vi "图像采集与保存-简单图像处理(加录像功能).vi"(9 "Grab":bool, 11 "Camera Name":refnum<k21>="cam0" caption="IMAQdx Session") -> ()   [LabVIEW 2022 SP3]
doc: "The Grab and Attributes Setup example VI allows the user to view the current attributes and settings, update attribute settings, acquire images continuously, and display the images in an image control."
uses:
  <vilib>/vision/Avi.llb/IMAQ AVI2 Refnum.ctl
  <vilib>/vision/driver/IMAQdx.llb/IMAQdx Acquisition Mode.ctl
  <vilib>/vision/driver/IMAQdx.llb/IMAQdx Buffer Number Mode.ctl
  <vilib>/vision/driver/NI_Vision_Acquisition_Software.lvlib
panel:
  in  "Boolean":bool
  out "视频路径":path
  out "time":u32
  out "Image 2":T1(plugin-control)
  out "AVI Refnum (duplicate)":T2
  out "millisecond timer value":u32
  out "AVI Refnum":T2
  in  "录制视频":bool
  out "Image out":T1(plugin-control)
  out "错误输出":errorcluster
  out "返回值":i32
  out "处理图片路径":path
  out "采集图片路径":path
  out "帧数":i32
  in  "采集帧间隔":i8
  in  "确定按钮":bool
  in  "Tab Control":T3(tab)
  in  "U32 Value Control":u32(slide) min=1 step=1 scale=1.0..4294967295.0
  in  "DBL Value Control":dbl(slide) min=2.2571161239684447 max=1000.0 step=1.0 scale=2.2571161239684447..1000.0
  in  "String Value Control":string
  in  "Enum Value Control":u32(ring) items=["Unicast", "Broadcast", "Multicast"]
  in  "Boolean Value Control":bool
  in  "Command Value Control":bool
  out "Tooltip":string="Gets/Sets the maximum number of outstanding events to queue."
  out "Units":string
  in  "Attribute Tree":string(tree)
  out "Frame Rate":dbl(knob) scale=0.0..100.0
  out "Image":T1(plugin-control)
  out "Buffer Number":u32
  in  "Stop":bool
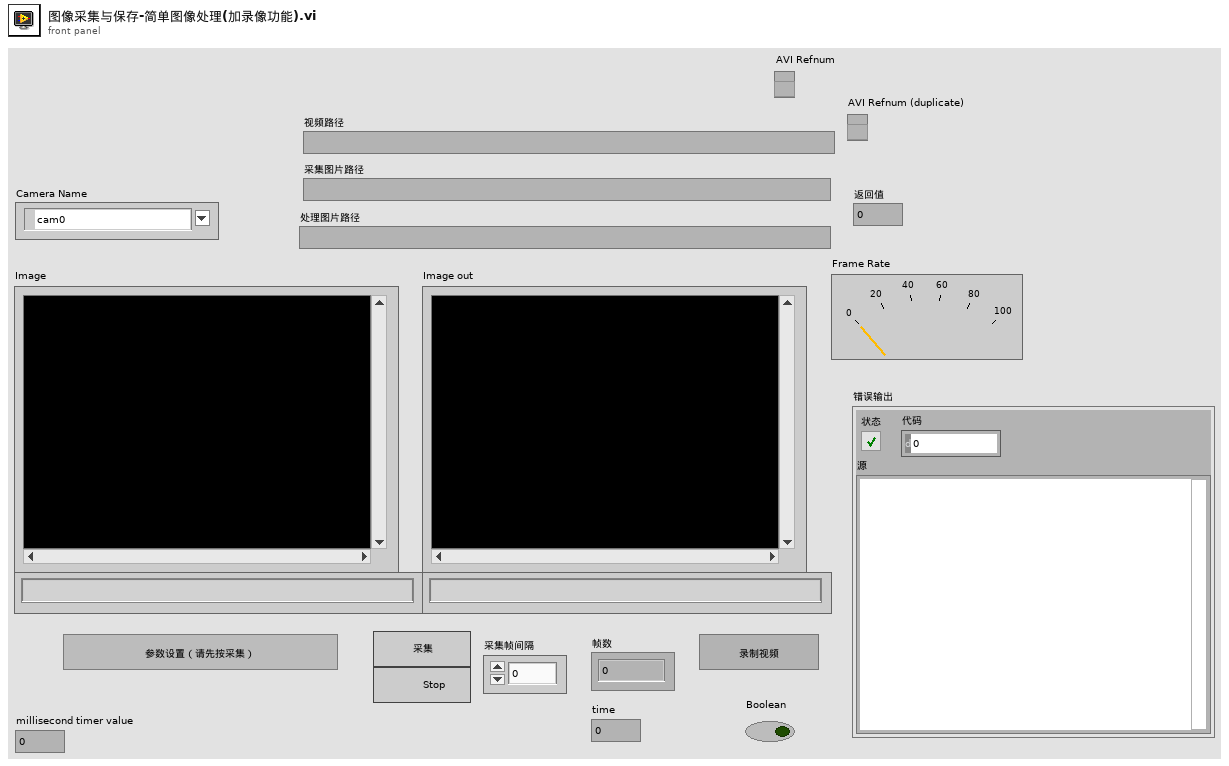
[diagram p1: front panel]
types:
  T1 = typedef "IMAQ Image.ctl" = refnum<image>
  T2 = typedef "IMAQ AVI2 Refnum.ctl" = refnum<k20>
  T3 = enum32{"U32", "DBL", "String", "Enum", "Bool", "Command"}
  T4 = typedef "NI_Vision_Acquisition_Software.lvlib/IMAQdx Acquisition Mode.ctl" = enum32{"One Shot", "Continuous"}
  T5 = typedef "IMAQdx.ctl" = refnum<k21>
  T6 = cluster{"Tab Control":refnum<vi>, "U32 Value Control":refnum<vi>, "DBL Value Control":refnum<vi>, "String Value Control":refnum<vi>, "Enum Value Control":refnum<vi>, "Boolean Value Control":refnum<vi>, "Command Value Control":refnum<vi>}
  T7 = typedef "NI_Vision_Acquisition_Software.lvlib/IMAQdx Buffer Number Mode.ctl" = enum32{"Next", "Last", "Buffer Number", "Every", "Last New"}
  T8 = typedef "Image Type" = u32
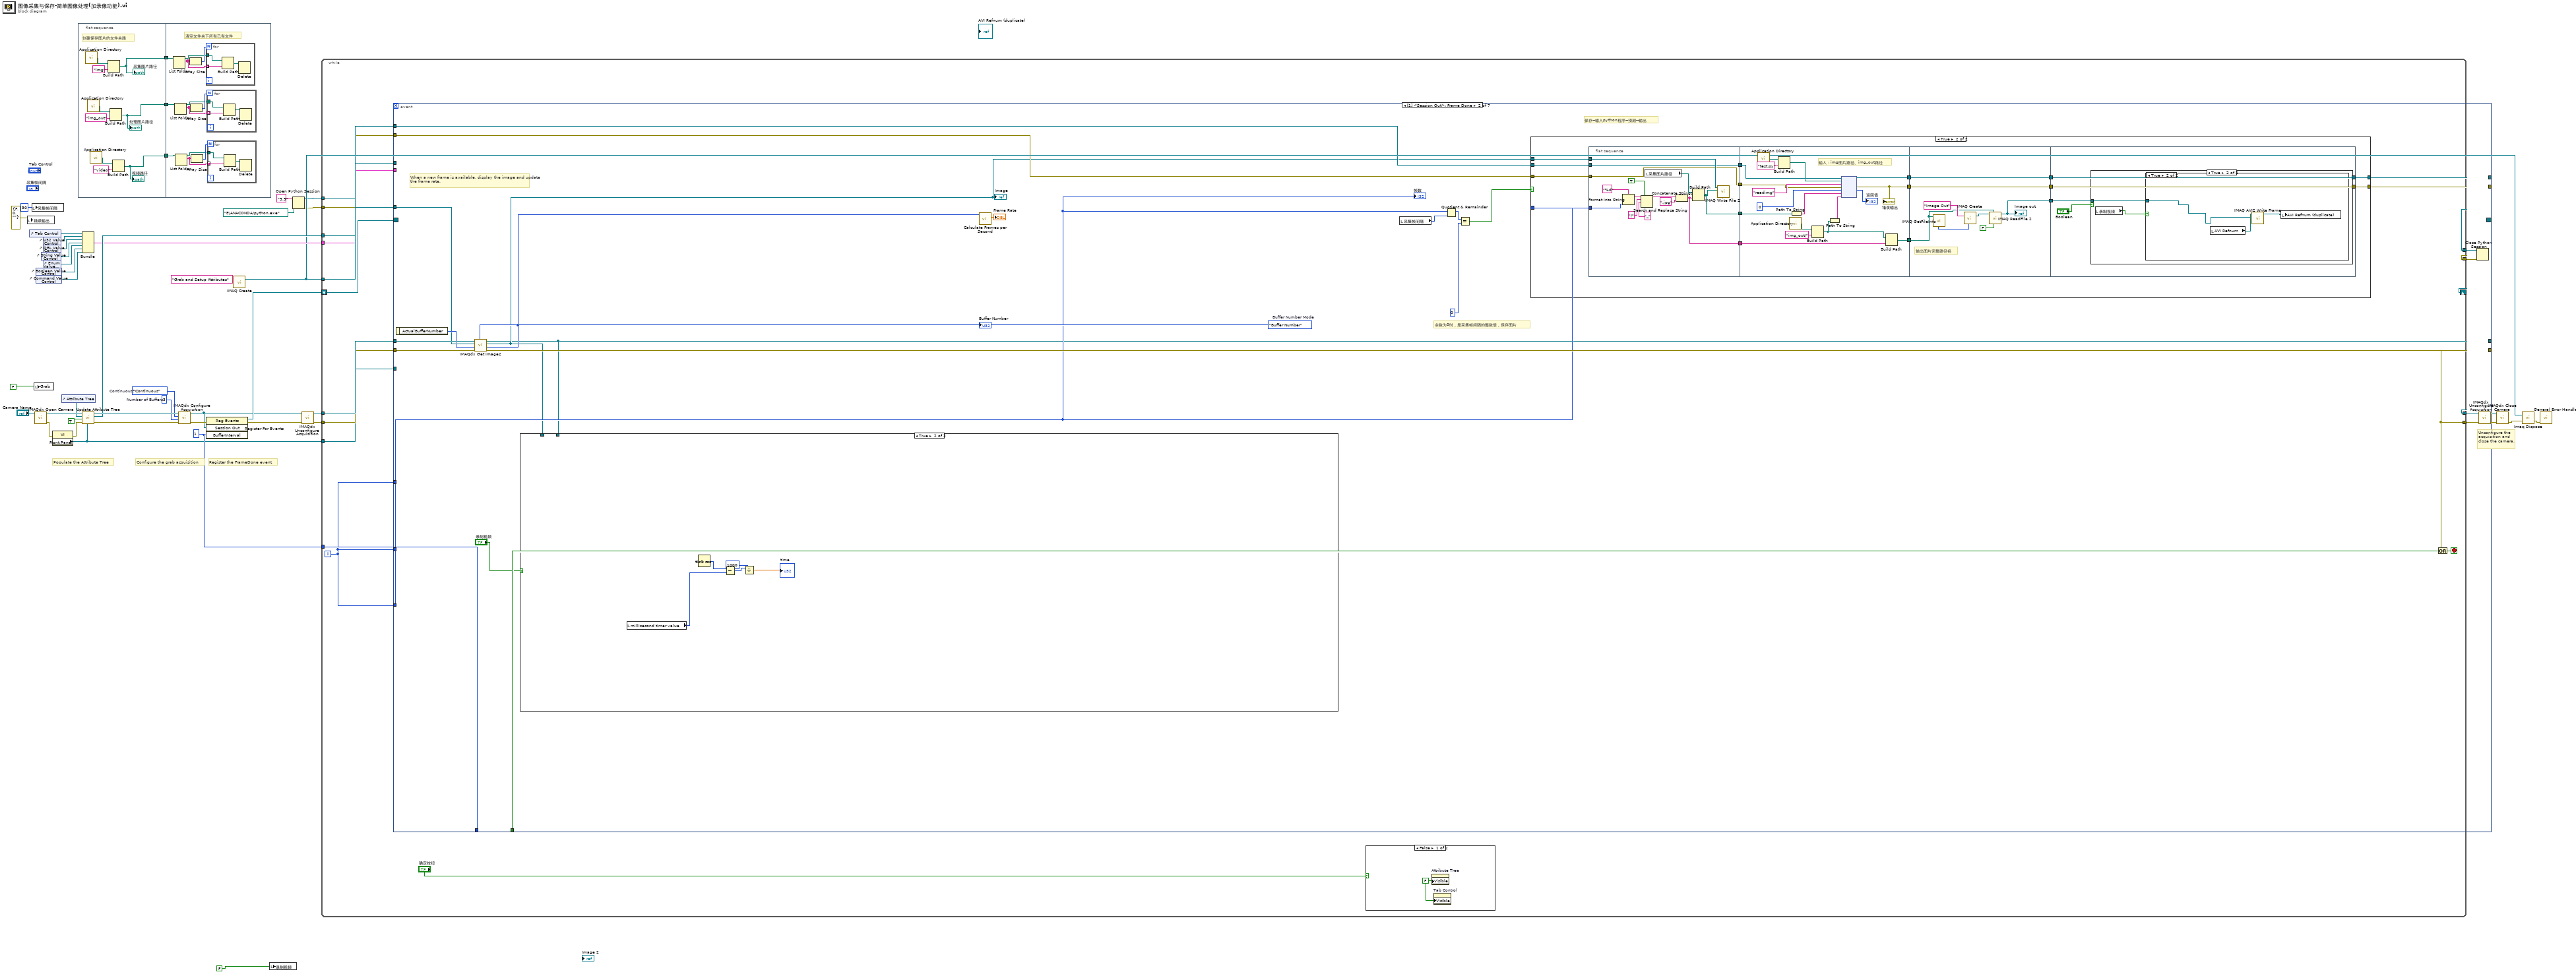
[diagram p0: block diagram]
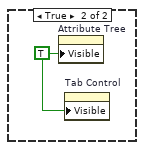
[diagram p2: hidden frame]
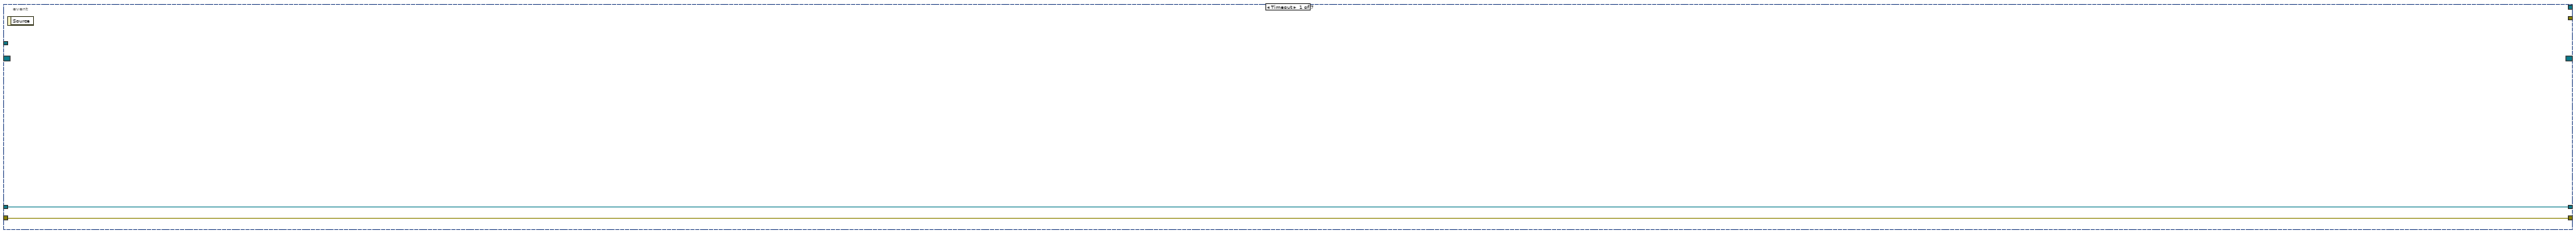
[diagram p3: hidden frame]
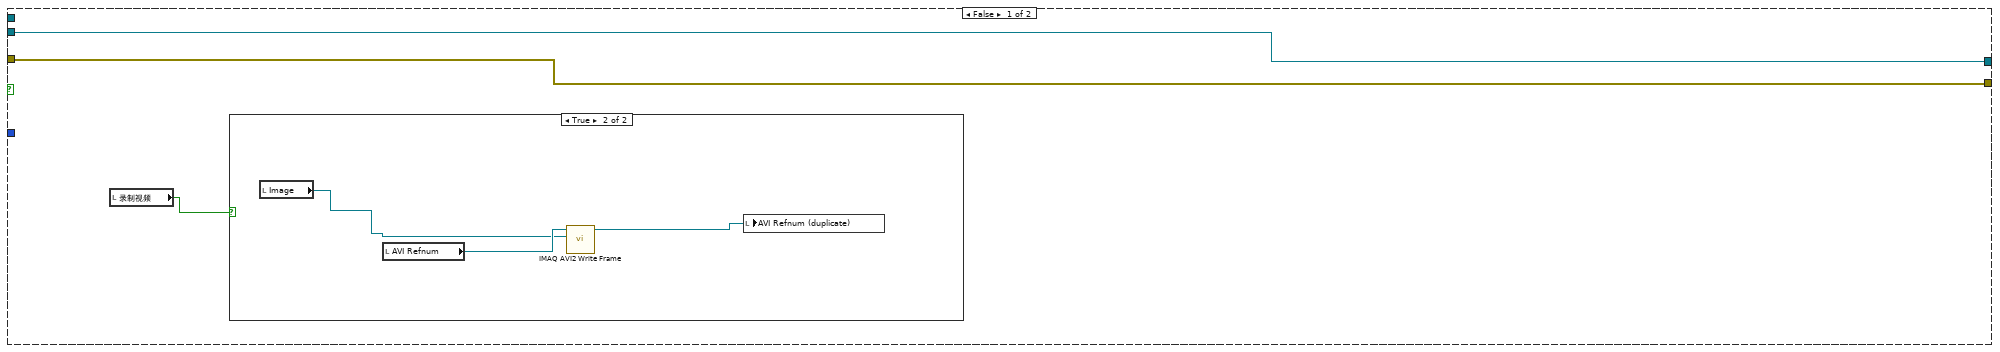
[diagram p5: hidden frame]
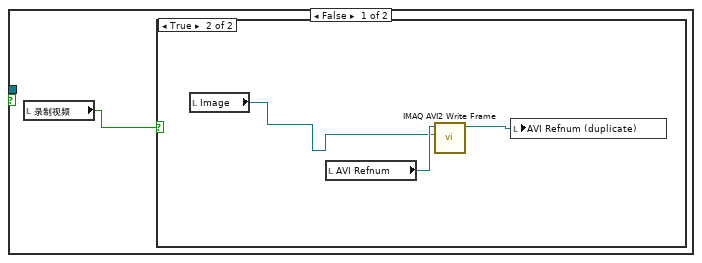
[diagram p7: hidden frame]
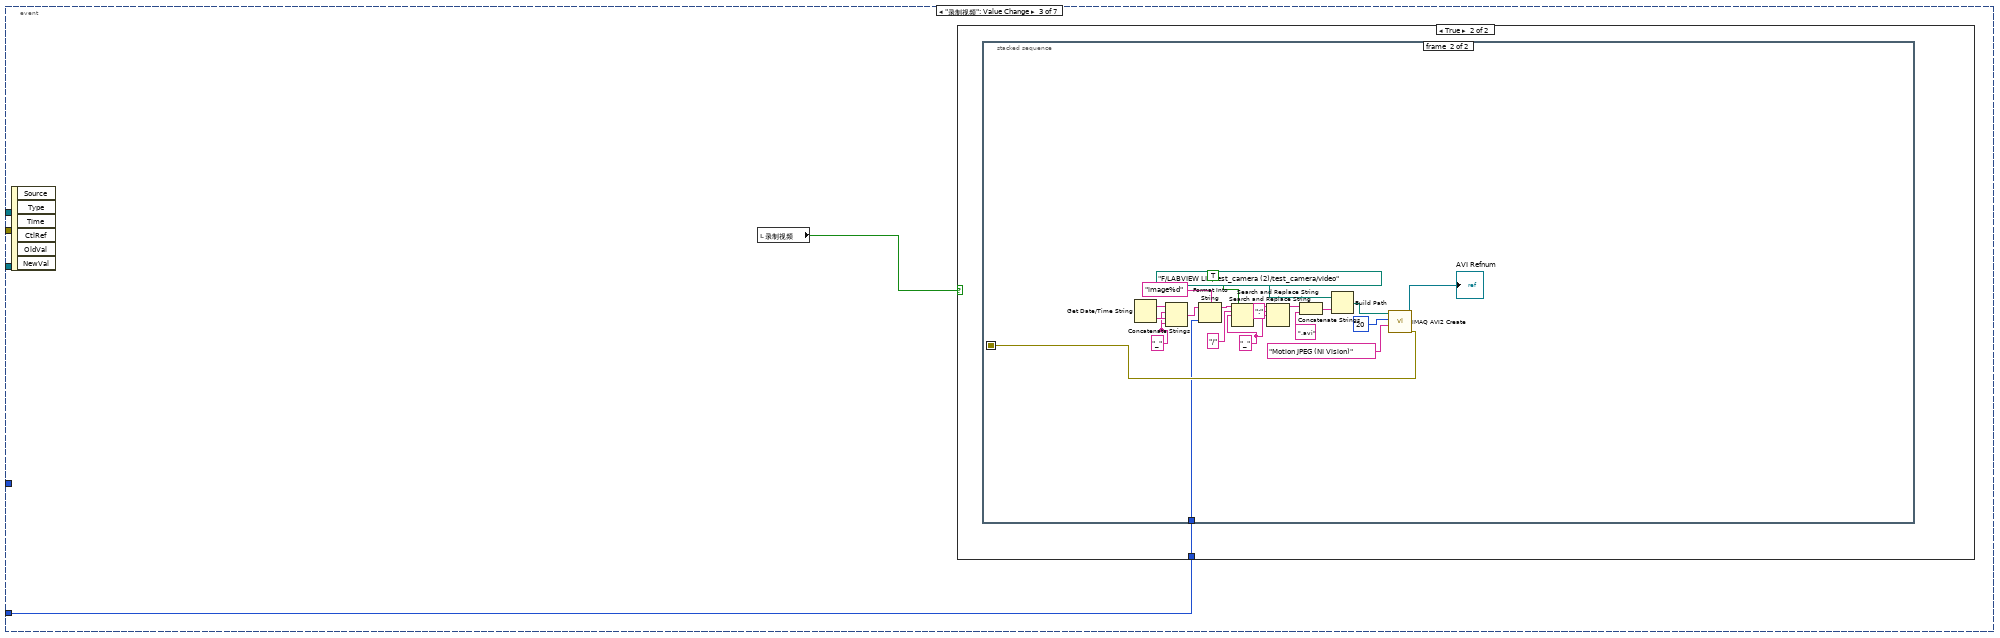
[diagram p10: hidden frame]
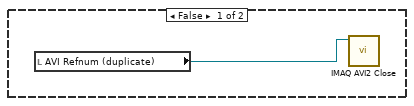
[diagram p11: hidden frame]
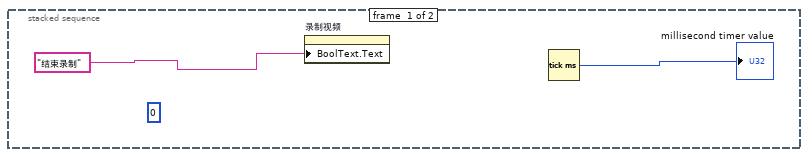
[diagram p12: hidden frame]
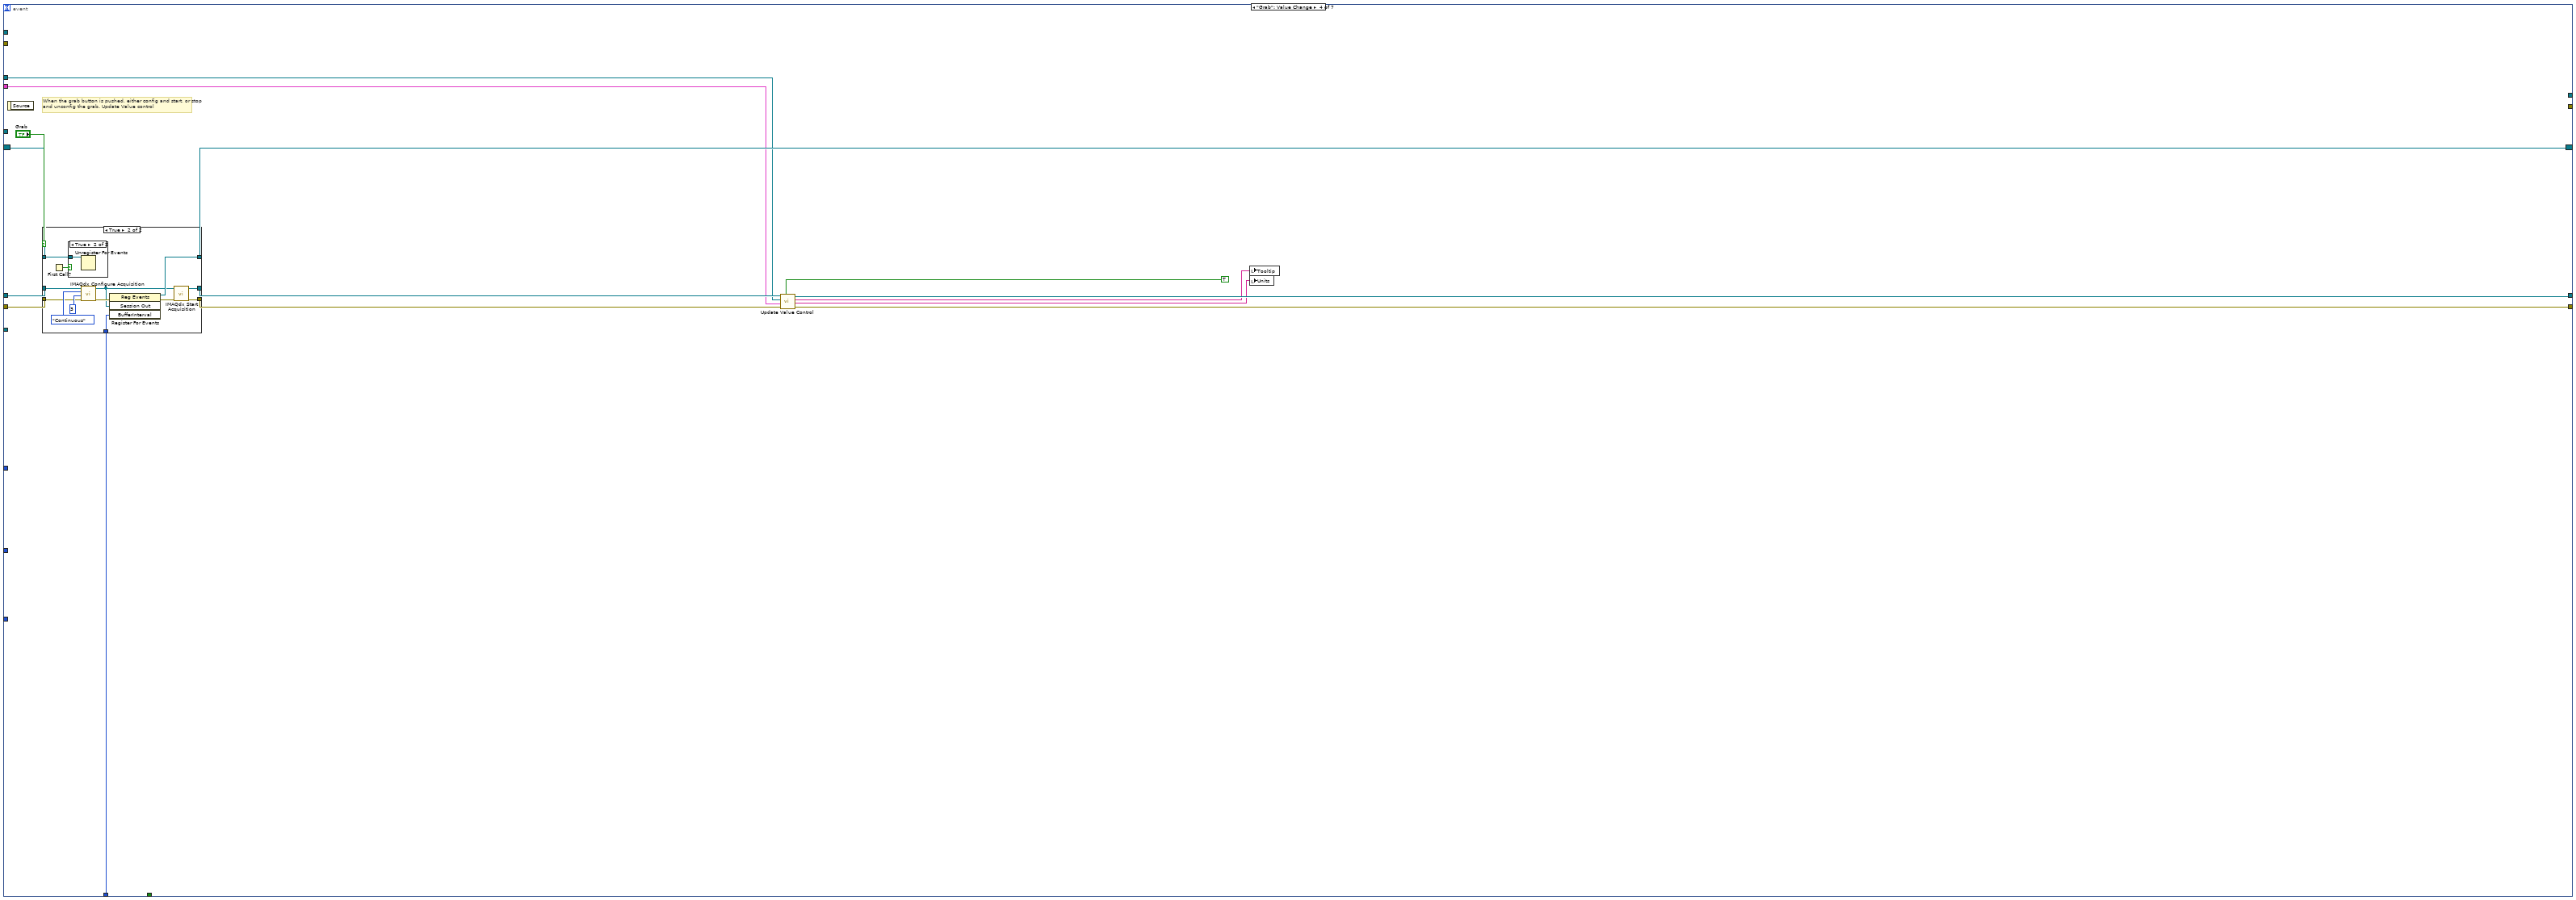
[diagram p13: hidden frame]
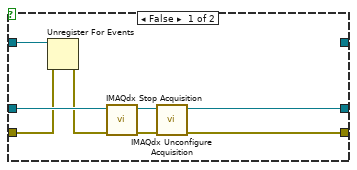
[diagram p14: hidden frame]
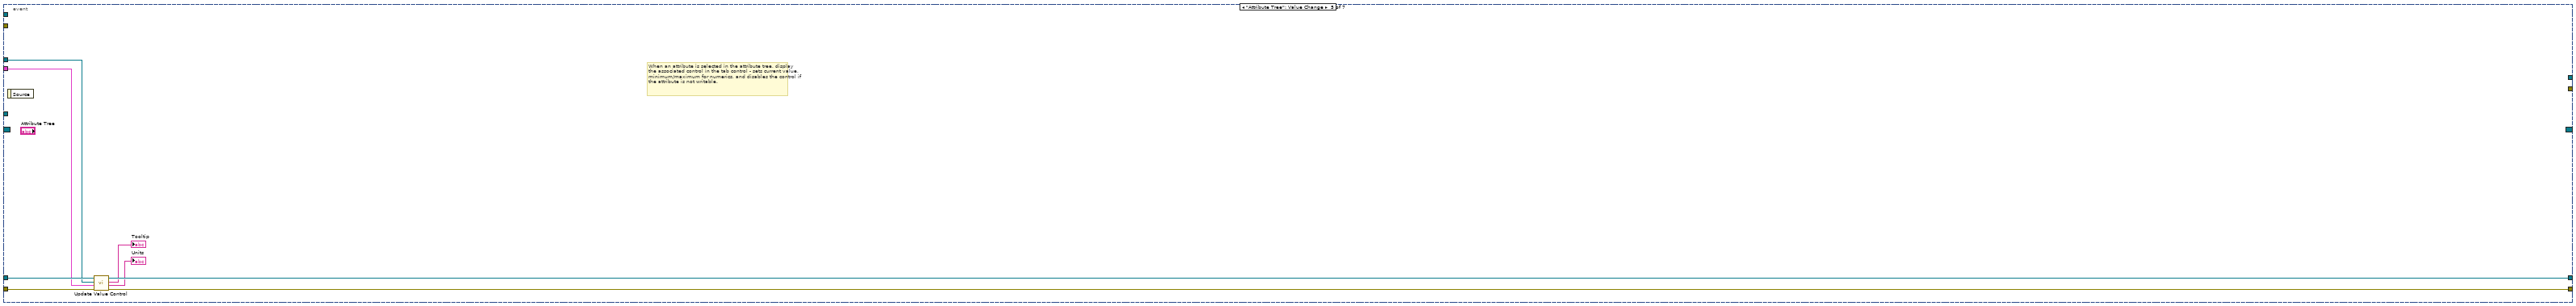
[diagram p16: hidden frame]
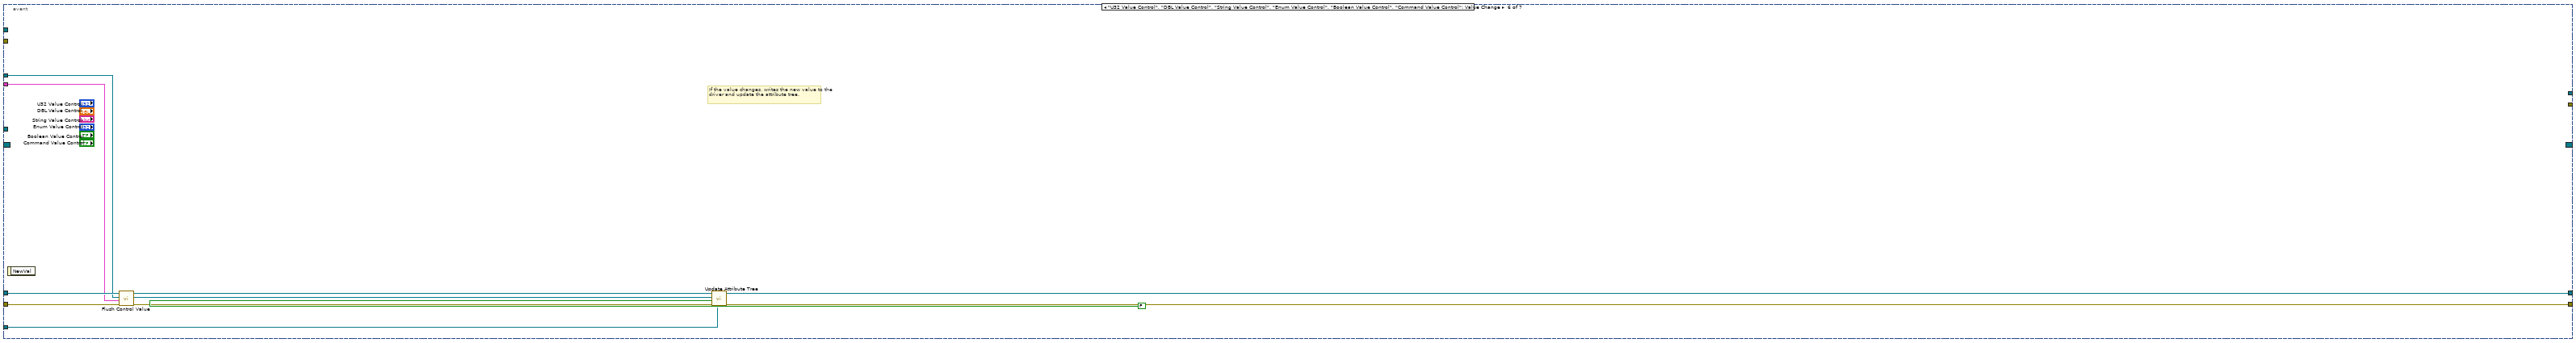
[diagram p17: hidden frame]
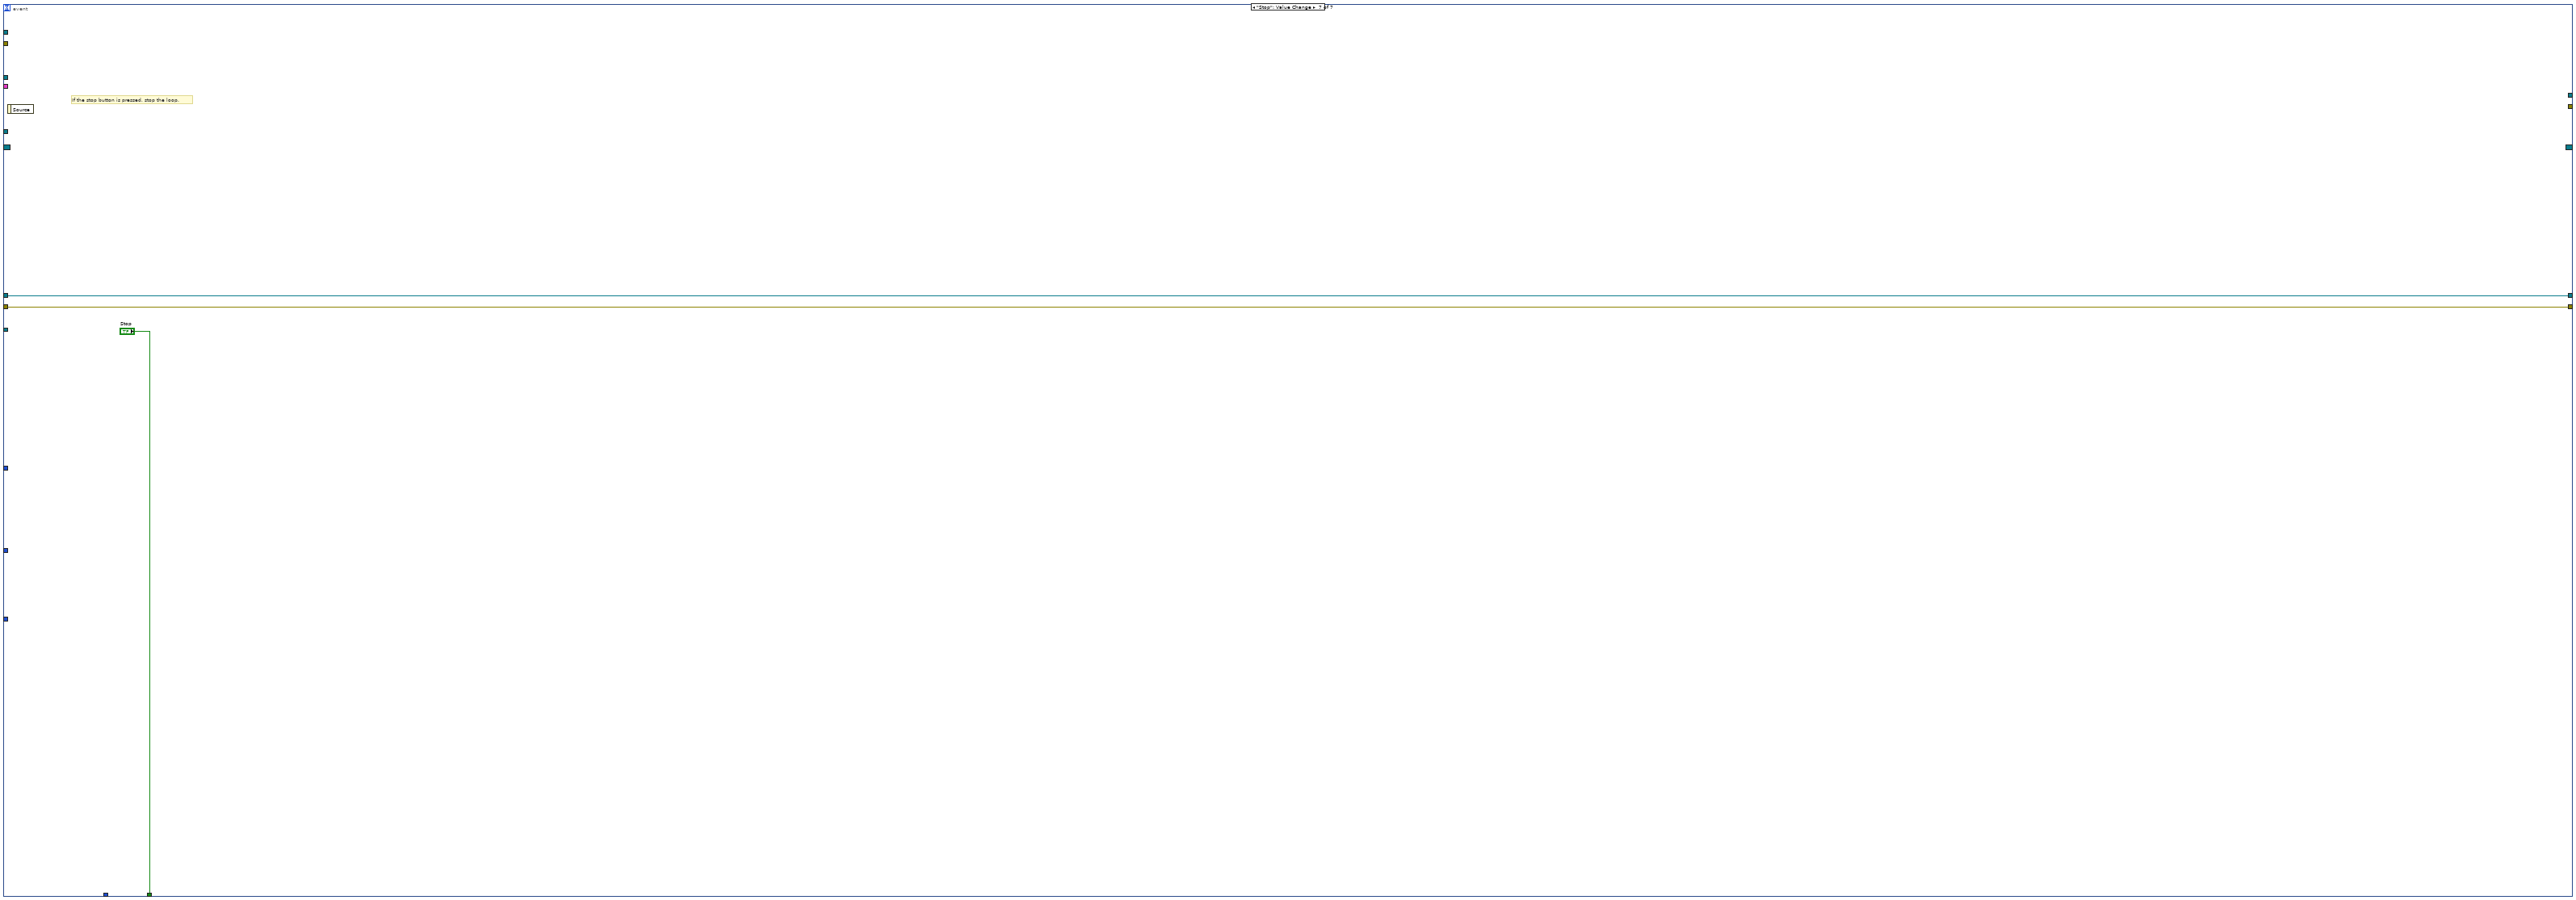
[diagram p18: hidden frame]
diagram:
  w29 = u32 1 ("BufferInterval")
  w15 = u32 3  # Number of Buffers
  w14 = IMAQdx_Acquisition_Mode."Continuous"  # Continuous?
  # "Unconfigure the acquisition and close the camera."
  # "Register the FrameDone event"
  # "Configure the grab acquisition"
  # "Populate the Attribute Tree"
  n1 = local write "错误输出"(errorcluster {"status"=FALSE, "code"=0, "source"=""} ("错误输出")) -> ()
  n2 = control-ref of="Tab Control"() -> (w19:refnum<vi>)
  n3 = local write "采集帧间隔"(i8 30 ("采集帧间隔")) -> ()
  n4 = local write "Grab"(FALSE ("Grab")) -> ()
  n5 = call <vilib>:"IMAQdx Open Camera.vi"("Session In"="Camera Name") -> ("error out"=w32:errorcluster, "Session Out"=w37:T5)  [unwired: 2 in, 7 out]
  n6 = control-ref of="Boolean Value Control"() -> (w39:refnum<vi>)
  n7 = control-ref of="Command Value Control"() -> (w38:refnum<vi>)
  n8 = control-ref of="String Value Control"() -> (w43:refnum<vi>)
  n9 = control-ref of="U32 Value Control"() -> (w42:refnum<vi>)
  n10 = control-ref of="DBL Value Control"() -> (w41:refnum<vi>)
  n11 = control-ref of="Enum Value Control"() -> (w40:refnum<vi>)
  n12 = property class="VI"(error in=w32) -> (error out=w18:errorcluster, "Front Panel"=w16:refnum<vi>)  [unwired: 1 in, 1 out]
  n13 = control-ref of="Attribute Tree"() -> (w35:refnum<vi>)
  n14 = flat-sequence {
    tunnel: [w55] -> w12
    tunnel: [w52] -> w10
    tunnel: [w49] -> w1
    tunnel: w12 -> [w66]
    tunnel: w10 -> [w62]
    tunnel: w1 -> [w58]
    frame #0 {
      # "创建保存图片的文件夹路"
      n15 = call <vilib>:"Application Directory.vi"() -> ("Application Directory"=w57:path)
      n16 = call <vilib>:"Application Directory.vi"() -> ("Application Directory"=w54:path)
      n17 = call <vilib>:"Application Directory.vi"() -> ("Application Directory"=w50:path)
      n18 = Build Path(base path=w57, name or relative path="img" ("名称或相对路径")) -> (appended path=w55:path)
      "采集图片路径" <- w55
      n19 = Build Path(base path=w54, name or relative path="img_out" ("名称或相对路径")) -> (appended path=w52:path)
      "处理图片路径" <- w52
      n20 = Build Path(base path=w50, name or relative path="video" ("名称或相对路径")) -> (appended path=w49:path)
      "视频路径" <- w49
    }
    frame #1 {
      # "清空文件夹下所有已有文件"
      n21 = List Folder(path=w66) -> (path out=w67:path, filenames=w69:string[])  [unwired: 3 in, 2 out]
      n22 = List Folder(path=w62) -> (path out=w63:path, filenames=w65:string[])  [unwired: 3 in, 2 out]
      n23 = List Folder(path=w58) -> (path out=w59:path, filenames=w61:string[])  [unwired: 3 in, 2 out]
      n24 = Array Size(array=w69) -> (size(s)=w68:i32)
      n25 = Array Size(array=w65) -> (size(s)=w64:i32)
      n26 = Array Size(array=w61) -> (size(s)=w60:i32)
      n27 = for {
        N: w68 -> [_]
        tunnel: w67 -> [w77]
        tunnel: w69 -> [w76] mode=indexing
        n28 = Build Path(base path=w77, name or relative path=w76) -> (appended path=w78:path)
        n29 = Delete(path (use dialog)=w78) -> ()  [unwired: 4 in, 3 out]
      }
      n30 = for {
        N: w64 -> [_]
        tunnel: w63 -> [w74]
        tunnel: w65 -> [w73] mode=indexing
        n31 = Build Path(base path=w74, name or relative path=w73) -> (appended path=w75:path)
        n32 = Delete(path (use dialog)=w75) -> ()  [unwired: 4 in, 3 out]
      }
      n33 = for {
        N: w60 -> [_]
        tunnel: w59 -> [w71]
        tunnel: w61 -> [w70] mode=indexing
        n34 = Build Path(base path=w71, name or relative path=w70) -> (appended path=w72:path)
        n35 = Delete(path (use dialog)=w72) -> ()  [unwired: 4 in, 3 out]
      }
    }
  }
  n36 = Bundle("Tab Control"=w19, "U32 Value Control"=w42, "DBL Value Control"=w41, "String Value Control"=w43, "Enum Value Control"=w40, "Boolean Value Control"=w39, "Command Value Control"=w38) -> (w24:T6)  [unwired: 1 out]
  n37 = call "Update Attribute Tree.vi"("Panel Refnum In"=w16, "error in"=w18, "Flush Tree?"=TRUE, "Tree Control In"=w35, "Camera Name In"=w37) -> ("error out"=w17:errorcluster, "Tree Control Out"=w33:refnum<vi>, "Session Out"=w36:T5)  [unwired: 4 in]
  n38 = call <vilib>:"IMAQdx Configure Acquisition.vi"("error in"=w17, "Number of Buffers"=w15, "Continuous?"=w14, "Session In"=w36) -> ("error out"=w45:errorcluster, "Session Out"=w26:T5)  [unwired: 6 out]
  n39 = register-events(error in=w45, w26, w29) -> (reference out=w44:refnum<event-registration>, error out=w28:errorcluster)  [unwired: 1 in]
  n40 = call "IMAQ Create"("Image Name"="Grab and Setup Attributes") -> ("New Image"=w21:T1)  [unwired: 3 in, 2 out]
  n41 = local write "录制视频"(FALSE) -> ()
  n42 = Open Python Session(python version="3.9" ("Python版本"), python path=path "E:/ANACONDA/python.exe" ("Python path")) -> (session out=w8:refnum<k35>, error out=w5:errorcluster)  [unwired: 1 in]
  n43 = call <vilib>:"IMAQdx Unconfigure Acquisition.vi"("error in"=w28, "Session In"=w26) -> ("error out"=w27:errorcluster, "Session Out"=w25:T5)  [unwired: 8 out]
  n44 = while {
    tunnel: [w93] -> w31
    tunnel: w27 -> [w95]
    tunnel: w25 -> [w96]
    tunnel: [w86] -> w30
    tunnel: w21 -> [w94]
    tunnel: w33 -> [w91]
    tunnel: w16 -> [w90]
    tunnel: w29 -> [w88]
    shift-right: [w87] -> _
    shift-left: w44 -> [w92]
    tunnel: w24 -> [w85]
    tunnel: w8 -> [w83]
    tunnel: [w82] -> w7
    tunnel: [w81] -> w6
    tunnel: w5 -> [w80]
    i -> [w79]
    stop <- w97 stop-if-true
    n45 = event shown="[1] <Session Out>: Frame Done" {
      selector: w92 -> [_ _ _ w239 _ _ _]
      dyn-events: [_ _ _ w241 _ _ _] -> w87
      timeout: _ -> [_ _ _ _ _ _ _]
      tunnel: w96 -> [w100 w121 _ w243 w273 w283 w285]
      tunnel: w95 -> [w101 w120 _ w238 w271 w284 w286]
      tunnel: w94 -> [_ w106 _ _ _ _ _]
      tunnel: [w100 w103 _ w231 w272 w279 w285] -> w93
      tunnel: [w101 w119 _ w235 w270 w275 w286] -> w86
      tunnel: w91 -> [_ _ _ w234 w268 w277 _]
      tunnel: w90 -> [_ _ _ _ _ w274 _]
      tunnel: [_ _ _ _ _ _ "Stop"] -> w89
      tunnel: w88 -> [_ _ _ w240 _ _ _]
      tunnel: w85 -> [_ _ _ w232 w269 w278 _]
      tunnel: w79 -> [_ w107 _ _ _ _ _]
      tunnel: w83 -> [_ w111 _ _ _ _ _]
      tunnel: [_ w110 _ _ _ _ _] -> w82
      tunnel: [_ w109 _ _ _ _ _] -> w81
      tunnel: w80 -> [_ w108 _ _ _ _ _]
      tunnel: w79 -> [_ _ _ _ _ _ _]
      tunnel: w79 -> [_ _ w203 _ _ _ _]
      event Timeout {
        n46 = event-data() -> ()  [unwired: 2 out]
      }
      event event #0x0 {
        w118 = IMAQdx_Buffer_Number_Mode."Buffer Number"  # Buffer Number Mode
        # "余数为0时，是采集帧间隔的整数倍，保存图片"
        # "保存--输入python程序--预测--输出"
        # "When a new frame is available, display the image and update the frame rate."
        n47 = event-data() -> ("ActualBufferNumber"=w117:u32)  [unwired: 1 out]
        n48 = call <vilib>:"IMAQdx Get Image2.vi"("Buffer Number Mode (Next)"=w118, "error in"=w120, "Buffer Number In"=w117, "Image In"=w106, "Session In"=w121) -> ("error out"=w119:errorcluster, "Buffer Number Out"=w116:u32, "Image Out"=w104:T1, "Session Out"=w103:T5)  [unwired: 3 in]
        "Image" <- w104
        "Buffer Number" <- w116
        n49 = case shown="True" "录制视频" {
          tunnel: w104 -> [_ _]
          tunnel: w103 -> [_ _]
          frame False {
          }
          frame True {
            n50 = local read "millisecond timer value"() -> (w125:u32)
            n51 = Tick Count (ms)() -> (millisecond timer value=w126:u32)
            n52 = Subtract(x=w126, y=w125) -> (x-y=w124:u32)
            n53 = Divide(x=w124, y=u32 1000) -> (x/y=→"time":dbl)
          }
        }
        n54 = call <vilib>:"Calculate Frames per Second.vi"("Buffer Number"=w116) -> ("Processed Frames/s"=→"Frame Rate":dbl)  [unwired: 8 in, 2 out]
        n55 = local read "采集帧间隔"() -> (w113:i8)
        n56 = Quotient & Remainder(x=w107, y=w113) -> (x-y*floor(x/y)=w112:i32)  [unwired: 1 out]
        n57 = Equal?(x=w112, y=i8 0) -> (x = y?=w102:bool)
        n58 = case shown="True" w102 {
          tunnel: w107 -> [_ w148]
          tunnel: w104 -> [_ w147]
          tunnel: w111 -> [w129 w145]
          tunnel: [w129 w143] -> w110
          tunnel: [w128 w142] -> w109
          tunnel: w108 -> [w128 w141]
          frame False {
            n59 = local read "录制视频"() -> (w127:bool)
            n60 = case shown="True" w127 {
              frame False {
              }
              frame True {
                n61 = local read "Image"() -> (w130:T1)
                n62 = local read "AVI Refnum"() -> (w131:T2)
                n63 = call "IMAQ AVI2 Write Frame"("Image"=w130, "AVI Refnum"=w131) -> ("AVI Refnum (duplicate)"=w132:T2)  [unwired: 7 in, 2 out]
                n64 = local write "AVI Refnum (duplicate)"(w132) -> ()
              }
            }
          }
          frame True {
            n65 = flat-sequence {
              tunnel: w148 -> [w155]
              tunnel: w147 -> [w154]
              tunnel: [w152] -> w146
              tunnel: w145 -> [w152]
              tunnel: [w151] -> w144
              tunnel: w141 -> [w150]
              tunnel: [w150] -> w140
              tunnel: [w149] -> w137
              tunnel: w146 -> [w180]
              tunnel: w144 -> [w174]
              tunnel: w140 -> [w169]
              tunnel: [w171] -> w139
              tunnel: [w170] -> w138
              tunnel: w137 -> [w164]
              tunnel: [w163] -> w136
              tunnel: w139 -> [w188]
              tunnel: w138 -> [w187]
              tunnel: w136 -> [w183]
              tunnel: [w188] -> w135
              tunnel: [w187] -> w134
              tunnel: [w181] -> w133
              tunnel: [w191] -> w142
              tunnel: [w192] -> w143
              tunnel: w135 -> [w192]
              tunnel: w134 -> [w191]
              tunnel: w133 -> [w189]
              frame #0 {
                n66 = Format Into String(format string="%d" ("Image Name"), w155) -> (resulting string=w156:string)  [unwired: 2 in, 1 out]
                n67 = Search and Replace String(replace all?=TRUE ("替换全部？(F)"), input string=w156, search string="/" ("搜索字符串"), replace string="_" ("替换字符串(\"\")")) -> (result string=w158:string)  [unwired: 4 in, 3 out]
                n68 = local read "采集图片路径"() -> (w153:path)
                n69 = Concatenate Strings(w158, ".jpg" ("字符串")) -> (w149:string)
                n70 = Build Path(base path=w153, name or relative path=w149) -> (appended path=w151:path)
                n71 = call-poly "IMAQ Write File 2"("File Path"=w151, "Image"=w154) -> ()  [unwired: 8 in, 2 out]
              }
              frame #1 {
                # "输入：img图片路径、img_out路径"
                n72 = call <vilib>:"Application Directory.vi"() -> ("Application Directory"=w179:path)
                n73 = Build Path(base path=w179, name or relative path="test.py" ("名称或相对路径")) -> (appended path=w177:path)
                n74 = call <vilib>:"Application Directory.vi"() -> ("Application Directory"=w168:path)
                n75 = Path To String(path=w174) -> (string=w173:string)
                n76 = Build Path(base path=w168, name or relative path="img_out/" ("名称或相对路径")) -> (appended path=w165:path)
                n77 = Path To String(path=w165) -> (string=w166:string)
                n78 = node(w180, w177, "readimg" ("函数名称"), w169, 0, w173, w166) -> (w171:refnum<k35>, w170:errorcluster, →"返回值":i32)  [unwired: 2 in, 2 out]
                "错误输出" <- w170
                n79 = Build Path(base path=w165, name or relative path=w164) -> (appended path=w163:path)
              }
              frame #2 {
                # "输出图片完整路径名"
                n80 = call "IMAQ GetFileInfo"("File Path"=w183) -> ("Image Type"=w182:T8)  [unwired: 4 in, 6 out]
                n81 = call "IMAQ Create"("Image Name"="Image Out", "Image Type"=w182) -> ("New Image"=w185:T1)  [unwired: 3 in, 1 out]
                n82 = call "IMAQ ReadFile 2"("Use File Path Image Type"=FALSE, "File Path"=w183, "Image"=w185) -> ("Image Out"=w181:T1)  [unwired: 4 in, 4 out]
                "Image out" <- w181
              }
              frame #3 {
                n83 = case shown="True" "Boolean" {
                  tunnel: w189 -> [_ w197]
                  frame False {
                    n84 = local read "录制视频"() -> (w193:bool)
                    n85 = case shown="True" w193 {
                      frame False {
                      }
                      frame True {
                        n86 = local read "Image"() -> (w194:T1)
                        n87 = local read "AVI Refnum"() -> (w195:T2)
                        n88 = call "IMAQ AVI2 Write Frame"("Image"=w194, "AVI Refnum"=w195) -> ("AVI Refnum (duplicate)"=w196:T2)  [unwired: 7 in, 2 out]
                        n89 = local write "AVI Refnum (duplicate)"(w196) -> ()
                      }
                    }
                  }
                  frame True {
                    n90 = local read "录制视频"() -> (w198:bool)
                    n91 = case shown="True" w198 {
                      tunnel: w197 -> [_ w199]
                      frame False {
                      }
                      frame True {
                        n92 = local read "AVI Refnum"() -> (w200:T2)
                        n93 = call "IMAQ AVI2 Write Frame"("Image"=w199, "AVI Refnum"=w200) -> ("AVI Refnum (duplicate)"=w201:T2)  [unwired: 7 in, 2 out]
                        n94 = local write "AVI Refnum (duplicate)"(w201) -> ()
                      }
                    }
                  }
                }
              }
            }
          }
        }
        "帧数" <- w107
      }
      event "录制视频": Value Change {
        n95 = event-data() -> ()  [unwired: 7 out]
        n96 = local read "录制视频"() -> (w202:bool)
        n97 = case shown="True" w202 {
          tunnel: w203 -> [_ w205]
          frame False {
            n98 = local read "AVI Refnum (duplicate)"() -> (w204:T2)
            n99 = call "IMAQ AVI2 Close"("AVI Refnum"=w204) -> ()  [unwired: 10 in, 1 out]
          }
          frame True {
            n100 = stacked-sequence {
              seq-local: [_ w216] -> [_ _]
              tunnel: w205 -> [_ w209]
              frame #0 {
                (unwired) u32 0 ("time")
                n101 = property on="录制视频" class="Bool (strict)"("BoolText.Text"="结束录制") -> ()  [unwired: 2 in, 2 out]
                n102 = Tick Count (ms)() -> (millisecond timer value=→"millisecond timer value":u32)
              }
              frame #1 {
                w214 = "_" ("替换字符串(\"\")")
                w213 = "_" ("替换字符串(\"\")")
                n103 = Get Date/Time String() -> (date string=w226:string, time string=w215:string)  [unwired: 3 in]
                n104 = Concatenate Strings(w226, w214, w215, w214) -> (w227:string)
                n105 = Format Into String(format string="image%d" ("Image Name"), initial string=w227, w209) -> (resulting string=w228:string)  [unwired: 1 in, 1 out]
                n106 = Search and Replace String(replace all?=TRUE ("替换全部？(F)"), input string=w228, search string="/" ("搜索字符串"), replace string=w213) -> (result string=w212:string)  [unwired: 4 in, 3 out]
                n107 = Search and Replace String(input string=w212, search string=":" ("搜索字符串"), replace string=w213) -> (result string=w211:string)  [unwired: 5 in, 3 out]
                n108 = Concatenate Strings(w211, ".avi" ("字符串")) -> (w225:string)
                n109 = Build Path(base path=path "F:/LABVIEW LIB/test_camera (2)/test_camera/video" ("基路径"), name or relative path=w225) -> (appended path=w218:path)
                n110 = call "IMAQ AVI2 Create"("Codec"="Motion JPEG (NI Vision)", "Frames Per Second"=u32 20, "AVI Path"=w218) -> ("error out"=w216:errorcluster, "AVI Refnum"=→"AVI Refnum":T2)  [unwired: 7 in]
              }
            }
          }
        }
      }
      event "Grab": Value Change {
        # "When the grab button is pushed, either config and start, or stop and unconfig the grab. Update Value control"
        n111 = event-data() -> ()  [unwired: 2 out]
        n112 = case shown="True" "Grab" {
          tunnel: w243 -> [w251 w262]
          tunnel: [w248 w264] -> w237
          tunnel: [w247 w263] -> w236
          tunnel: [_ w257] -> w241
          tunnel: w240 -> [_ w255]
          tunnel: w239 -> [w246 w253]
          tunnel: w238 -> [w244 w254]
          frame False {
            n113 = Unregister For Events(event registration refnum=w246, error in=w244) -> (error out=w245:errorcluster)
            n114 = call <vilib>:"IMAQdx Stop Acquisition.vi"("error in"=w245, "Session In"=w251) -> ("error out"=w249:errorcluster, "Session Out"=w250:T5)  [unwired: 8 out]
            n115 = call <vilib>:"IMAQdx Unconfigure Acquisition.vi"("error in"=w249, "Session In"=w250) -> ("error out"=w247:errorcluster, "Session Out"=w248:T5)  [unwired: 8 out]
          }
          frame True {
            n116 = First Call?() -> (First Call?: T/F=w252:bool)
            n117 = case shown="True" w252 {
              tunnel: w253 -> [_ w265]
              frame False {
              }
              frame True {
                n118 = Unregister For Events(event registration refnum=w265) -> ()  [unwired: 1 in, 1 out]
              }
            }
            n119 = call <vilib>:"IMAQdx Configure Acquisition.vi"("error in"=w254, "Number of Buffers"=u32 3, "Continuous?"=IMAQdx_Acquisition_Mode."Continuous", "Session In"=w262) -> ("error out"=w259:errorcluster, "Session Out"=w256:T5)  [unwired: 6 out]
            n120 = register-events(error in=w259, w256, w255) -> (reference out=w257:refnum<event-registration>, error out=w258:errorcluster)  [unwired: 1 in]
            n121 = call <vilib>:"IMAQdx Start Acquisition.vi"("error in"=w258, "Session In"=w256) -> ("error out"=w263:errorcluster, "Session Out"=w264:T5)  [unwired: 8 out]
          }
        }
        n122 = call "Update Value Control.vi"("Force update?"=TRUE, "error in (no error)"=w236, "Tab Control Ref In"=w232, "Tree Control In"=w234, "Session In"=w237) -> ("error out"=w235:errorcluster, "Units"=w229:string, "Tooltip"=w230:string, "Session Out"=w231:T5)  [unwired: 3 in]
        n123 = local write "Tooltip"(w230) -> ()
        n124 = local write "Units"(w229) -> ()
      }
      event "Attribute Tree": Value Change {
        # "When an attribute is selected in the attribute tree, display the associated control in the tab control - sets current value, minimum/maximum for numerics, and disables the control if the attribute is not writable."
        n125 = event-data() -> ()  [unwired: 2 out]
        n126 = call "Update Value Control.vi"("error in (no error)"=w271, "Tab Control Ref In"=w269, "Tree Control In"=w268, "Session In"=w273) -> ("error out"=w270:errorcluster, "Units"=→"Units":string, "Tooltip"=→"Tooltip":string, "Session Out"=w272:T5)  [unwired: 4 in]
      }
      event "U32 Value Control", "DBL Value Control", "String Value Control", "Enum Value Control", "Boolean Value Control", "Command Value Control": Value Change {
        # "If the value changes, writes the new value to the driver and update the attribute tree."
        n127 = event-data() -> ()  [unwired: 2 out]
        n128 = call "Flush Control Value.vi"("error in (no error)"=w284, "Tab Control Ref In"=w278, "Tree Control In"=w277, "Session In"=w283) -> ("error out"=w276:errorcluster, "Tree Control Out"=w281:refnum<vi>, "Session Out"=w282:T5)  [unwired: 5 in]
        n129 = call "Update Attribute Tree.vi"("Panel Refnum In"=w274, "error in"=w276, "Flush Tree?"=FALSE, "Tree Control In"=w281, "Camera Name In"=w282) -> ("error out"=w275:errorcluster, "Session Out"=w279:T5)  [unwired: 4 in, 1 out]
      }
      event "Stop": Value Change {
        # "If the stop button is pressed, stop the loop."
        n130 = event-data() -> ()  [unwired: 2 out]
      }
    }
    n131 = case shown="False" "确定按钮" {
      frame False {
        w98 = FALSE ("可见")
        n132 = property on="Attribute Tree" class="Tree (strict)"("Visible"=w98) -> ()  [unwired: 2 in, 2 out]
        n133 = property on="Tab Control" class="TabCtl (strict)"("Visible"=w98) -> ()  [unwired: 2 in, 2 out]
      }
      frame True {
        w99 = TRUE ("可见")
        n134 = property on="Attribute Tree" class="Tree (strict)"("Visible"=w99) -> ()  [unwired: 2 in, 2 out]
        n135 = property on="Tab Control" class="TabCtl (strict)"("Visible"=w99) -> ()  [unwired: 2 in, 2 out]
      }
    }
    n136 = Or(x=w86, y=w89) -> (x .or. y?=w97:bool)
  }
  n137 = Close Python Session(session in=w7, error in=w6) -> ()  [unwired: 1 out]
  n138 = call <vilib>:"IMAQdx Unconfigure Acquisition.vi"("error in"=w30, "Session In"=w31) -> ("error out"=w47:errorcluster, "Session Out"=w46:T5)  [unwired: 8 out]
  n139 = call <vilib>:"IMAQdx Close Camera.vi"("error in"=w47, "Session In"=w46) -> ("error out"=w23:errorcluster)  [unwired: 9 out]
  n140 = call "Imaq Dispose"("Image"=w21, "error in (no error)"=w23) -> ("error out"=w22:errorcluster)  [unwired: 4 in]
  n141 = call <vilib>:"General Error Handler.vi"("error in (no error)"=w22) -> ()  [unwired: 2 in, 13 out]
